vi "range for XY graf.vi"(10 "range":dbl=3600.0, 11 "XY Graf":cluster{timestamp[], dbl[]}[](array[cluster])) -> (2 "start time":timestamp, 3 "end time":timestamp)   [LabVIEW 2019, in "Userlib.lvlib"]
uses:
  Userlib.lvlib
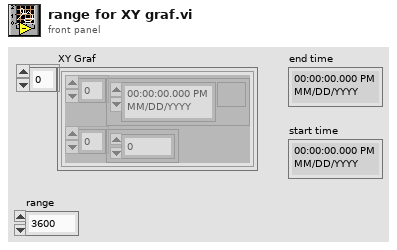
[diagram p1: front panel]
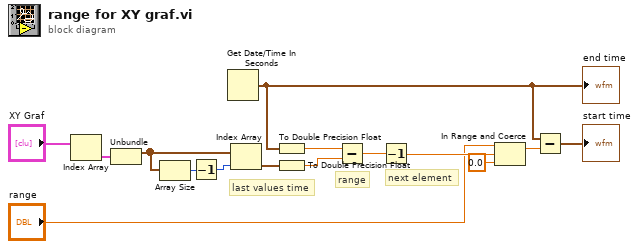
[diagram p0: block diagram]
diagram:
  # "range"
  # "next element"
  # "last values time"
  n1 = Index Array(array="XY Graf") -> (element=w6:cluster{timestamp[], dbl[]})  [unwired: 1 in]
  n2 = Unbundle(w6) -> (w8:timestamp[])  [unwired: 1 out]
  n3 = Array Size(array=w8) -> (size(s)=w7:i32)
  n4 = Decrement(x=w7) -> (x-1=w9:i32)
  n5 = Get Date/Time In Seconds() -> (seconds since 1Jan1904=w12:timestamp)
  "end time" <- w12
  n6 = Index Array(array=w8, index=w9) -> (element=w10:timestamp)
  n7 = To Double Precision Float(number=w12) -> (double precision float=w11:dbl)
  n8 = To Double Precision Float(number=w10) -> (double precision float=w5:dbl)
  n9 = Subtract(x=w11, y=w5) -> (x-y=w13:dbl)
  n10 = Decrement(x=w13) -> (x-1=w4:dbl)
  n11 = In Range and Coerce(upper limit="range", x=w4, lower limit=0.0) -> (coerced(x)=w1:dbl)  [unwired: 1 out]
  n12 = Subtract(x=w12, y=w1) -> (x-y=→"start time":timestamp)
